vi "Spatial Dual Decode Packet 37 (SubVI).vi"(8 "SGL Precision":i16=6, 10 "Packet 37 Bytes In":u8[](array[numeric])) -> (0 "Channel Data Type":string[](array[string])=["Float", "Float", "Float"], 1 "Channel Units":string[](array[string])=["m/s/s", "m/s/s", "m/s/s"], 2 "Data":string[](array[string]), 3 "Channel Names":string[](array[string])=["Acc X", "Acc Y", "Acc Z"], 4 "Packet 37 Decoded Data Cluster":T1)   [LabVIEW 2019, in "SpatialDual_Parsers.lvlib"]
uses:
  SpatialDual_Parsers.lvlib
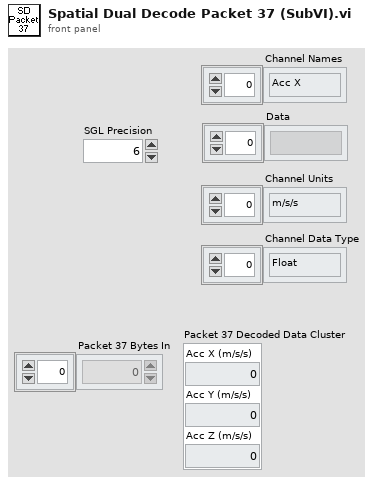
[diagram p1: front panel]
types:
  T1 = cluster{"Acc X (m/s/s)":sgl, "Acc Y (m/s/s)":sgl, "Acc Z (m/s/s)":sgl}
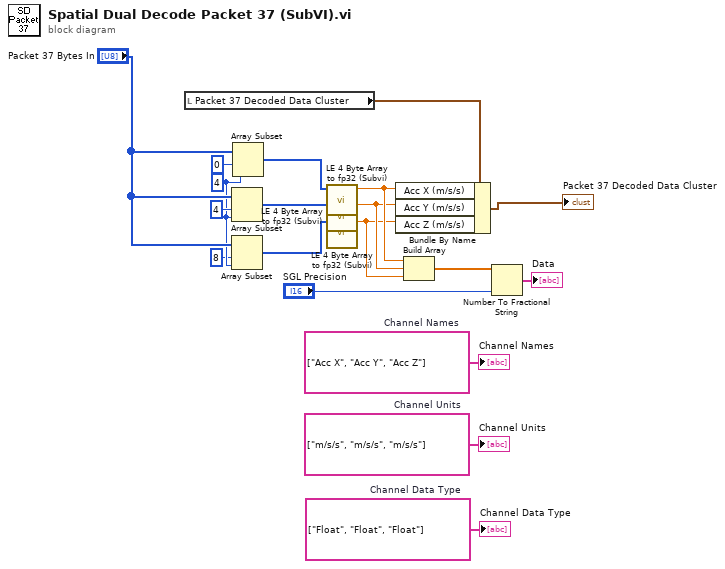
[diagram p0: block diagram]
diagram:
  w1 = string[] ["Float", "Float", "Float"]  # Channel Data Type
  w2 = string[] ["m/s/s", "m/s/s", "m/s/s"]  # Channel Units
  w3 = string[] ["Acc X", "Acc Y", "Acc Z"]  # Channel Names
  w14 = 4 ("length")
  n1 = local read "Packet 37 Decoded Data Cluster"() -> (w19:T1)
  n2 = Array Subset(array="Packet 37 Bytes In", index=4, length=w14) -> (w11:u8[])
  n3 = Array Subset(array="Packet 37 Bytes In", index=8, length=w14) -> (w12:u8[])
  n4 = Array Subset(array="Packet 37 Bytes In", index=0, length=w14) -> (w10:u8[])
  n5 = call "LE 4 Byte Array to fp32 (Subvi).vi"("4 Bytes in"=w10) -> ("fp32 Out"=w9:sgl)  [unwired: 8 in]
  n6 = call "LE 4 Byte Array to fp32 (Subvi).vi"("4 Bytes in"=w11) -> ("fp32 Out"=w8:sgl)  [unwired: 8 in]
  n7 = call "LE 4 Byte Array to fp32 (Subvi).vi"("4 Bytes in"=w12) -> ("fp32 Out"=w7:sgl)  [unwired: 8 in]
  n8 = Bundle By Name(cluster=w19, "Acc X (m/s/s)"=w9, "Acc Y (m/s/s)"=w8, "Acc Z (m/s/s)"=w7) -> (→"Packet 37 Decoded Data Cluster":T1)
  n9 = Build Array(w9, w8, w7) -> (w6:sgl[])
  n10 = Number To Fractional String(number=w6, precision (6)="SGL Precision") -> (F-format string=→"Data":string[])  [unwired: 2 in]
  "Channel Names" <- w3
  "Channel Units" <- w2
  "Channel Data Type" <- w1
